vi "Prober_ThetaAlignment.vi"(4 "y2":i32, 5 "y1":i32, 6 "x2":i32, 7 "x1":i32, 8 "error in (no error)":errorcluster, 11 "ProbeStationControl in":refnum<class "ProbeStationControl.lvclass">) -> (0 "error out":errorcluster, 1 "theta increment":i32, 2 "New millidegrees":i32, 3 "ProbeStationControl out":refnum<class "ProbeStationControl.lvclass">)   [LabVIEW 2019, in "ProbeStationControl.lvclass"]
uses:
  ProbeStationControl.lvclass
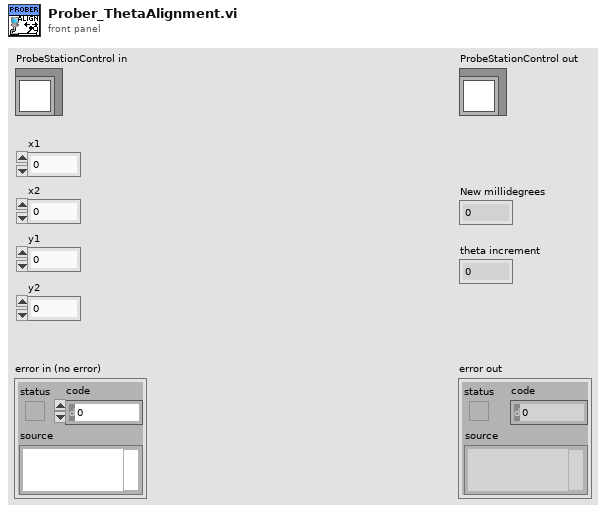
[diagram p1: front panel]
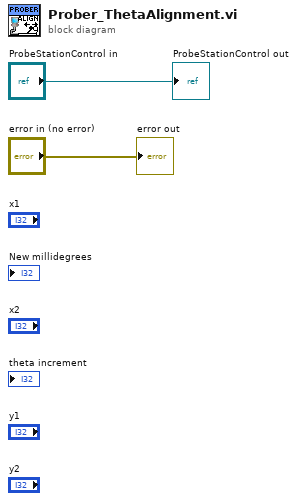
[diagram p0: block diagram]
diagram:
  "error out" <- "error in (no error)"
  "ProbeStationControl out" <- "ProbeStationControl in"
